vi "Open Panel TK.vi"(8 "error in (no error)":errorcluster, 10 "use VI Setup settings? (T)":bool=TRUE, 11 "VI name":string) -> (0 "error out":errorcluster)   [LabVIEW 2012]
doc: "Opens the panel of the specified VI. The specified VI must already be in memory, either because it was loaded using the Preload Instrument VI, or because it is the subVI of another VI."
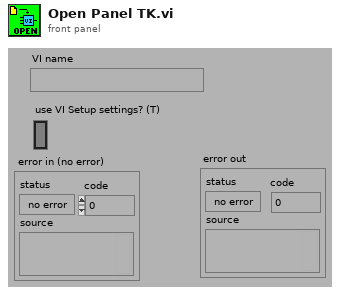
[diagram p1: front panel]
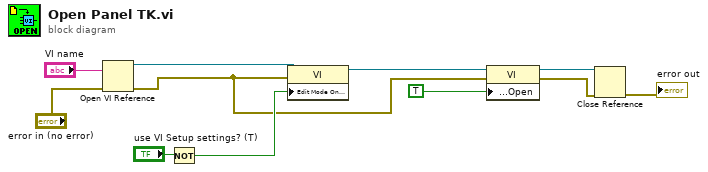
[diagram p0: block diagram]
diagram:
  n1 = Open VI Reference(vi path="VI name", error in (no error)="error in (no error)") -> (vi reference=w6:refnum<vi>, error out=w1:errorcluster)  [unwired: 4 in]
  n2 = Not(x="use VI Setup settings? (T)") -> (.not. x?=w8:bool)
  n3 = property class="VI"(reference=w6, error in=w1, "Edit Mode On Open"=w8) -> (reference out=w5:refnum<vi>)  [unwired: 1 out]
  n4 = property class="VI"(reference=w5, error in=w1, "Front Panel Window:Open"=TRUE) -> (reference out=w4:refnum<vi>, error out=w3:errorcluster)
  n5 = Close Reference(reference=w4, error in (no error)=w3) -> (error out=→"error out":errorcluster)
